vi "STS Calculator-File.vi"(6 "Hysteresis Analysis":enum32{"1st Sweep", "2nd Sweep", "Both"}(radio), 8 "NumPts":i32=3, 9 "Vd_Lin Index":i32, 10 "Vd_Sat Index":i32, 11 "Path":path) -> (0 "Used Points":T1, 1 "XY Graph-Sat":cluster{dbl[], dbl[]}[](graph), 2 "XY Graph-Lin":cluster{dbl[], dbl[]}[](graph), 3 "Ouput":cluster{"STS-Sat":dbl, "STS-Lin":dbl})   [LabVIEW 2012]
uses:
  <vilib>/Utility/file.llb/Read From Spreadsheet File (string).vi
panel:
  out "STS-Lin":dbl
  out "Linear Id":dbl[](array[numeric])
  out "Saturation Id":dbl[](array[numeric])
  out "Vg Column":dbl[](array[numeric])
  out "STS-Sat":dbl
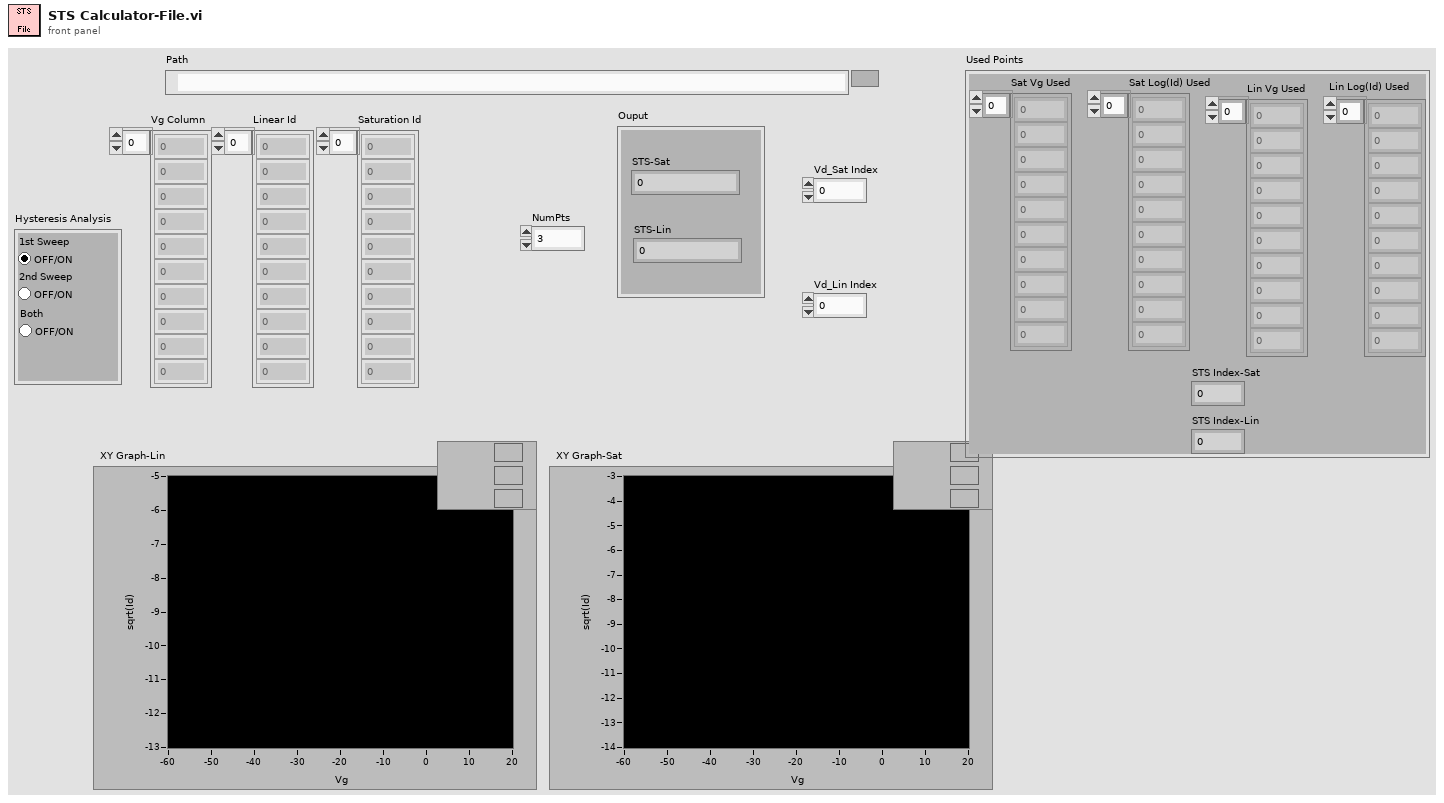
[diagram p1: front panel]
types:
  T1 = cluster{"Sat Vg Used":dbl[], "Sat Log(Id) Used":dbl[], "Lin Vg Used":dbl[], "Lin Log(Id) Used":dbl[], "STS Index-Sat":dbl, "STS Index-Lin":dbl}
  T2 = cluster{"Sub Threshold Swing":dbl, "Sub Threshold Swing":dbl}
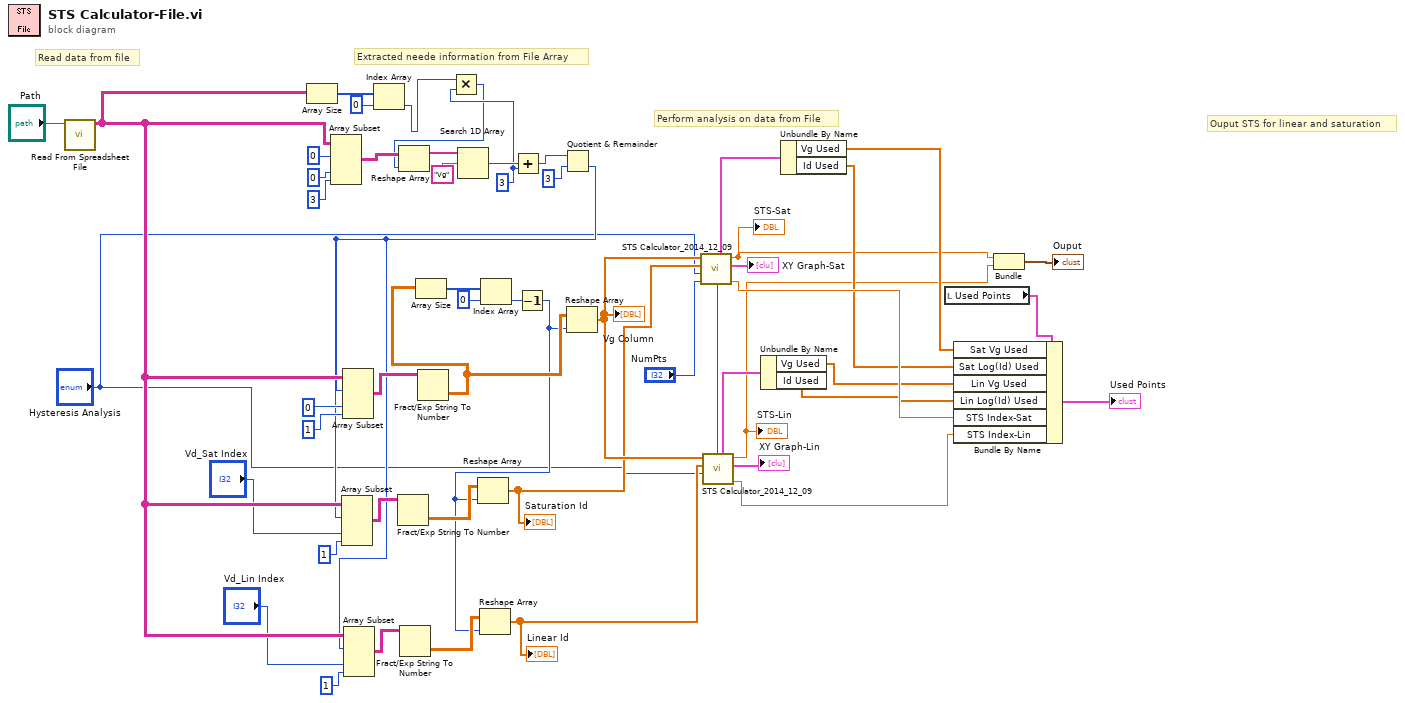
[diagram p0: block diagram]
diagram:
  w7 = 3
  # "Ouput STS for linear and saturation"
  # "Read data from file"
  # "Extracted neede information from File Array"
  # "Perform analysis on data from File"
  n1 = call-poly <vilib>:"Read From Spreadsheet File.vi"("file path (dialog if empty)"="Path") -> ("all rows"=w17:string[][])  [unwired: 6 in, 4 out]
  n2 = Array Size(array=w17) -> (size(s)=w28:i32[])
  n3 = Array Subset(array=w17, index (row)=0, index (col)=0, length (col)=3) -> (w40:string[][])  [unwired: 1 in]
  n4 = Index Array(array=w28, index=0) -> (element=w6:i32)
  n5 = Multiply(x=w6, y=w7) -> (x*y=w5:i32)
  n6 = Reshape Array(w40, w5) -> (w41:string[])
  n7 = Search 1D Array(1D array=w41, element="Vg") -> (index of element=w35:i32)  [unwired: 1 in]
  n8 = Add(x=w35, y=w7) -> (x+y=w10:i32)
  n9 = Quotient & Remainder(x=w10, y=3) -> (floor(x/y)=w8:i32)  [unwired: 1 out]
  n10 = Array Subset(array=w17, index (row)=w8, index (col)="Vd_Sat Index", length (col)=1) -> (w30:string[][])  [unwired: 1 in]
  n11 = Array Subset(array=w17, index (row)=w8, index (col)=0, length (col)=1) -> (w31:string[][])  [unwired: 1 in]
  n12 = Array Subset(array=w17, index (row)=w8, index (col)="Vd_Lin Index", length (col)=1) -> (w21:string[][])  [unwired: 1 in]
  n13 = Fract/Exp String To Number(string=w30) -> (number=w23:dbl[][])  [unwired: 3 in, 1 out]
  n14 = Fract/Exp String To Number(string=w21) -> (number=w22:dbl[][])  [unwired: 3 in, 1 out]
  n15 = Fract/Exp String To Number(string=w31) -> (number=w24:dbl[][])  [unwired: 3 in, 1 out]
  n16 = Array Size(array=w24) -> (size(s)=w27:i32[])
  n17 = Index Array(array=w27, index=0) -> (element=w25:i32)
  n18 = Decrement(x=w25) -> (x-1=w19:i32)
  n19 = Reshape Array(w23, w19) -> (w14:dbl[])
  "Saturation Id" <- w14
  n20 = Reshape Array(w22, w19) -> (w13:dbl[])
  "Linear Id" <- w13
  n21 = Reshape Array(w24, w19) -> (w15:dbl[])
  "Vg Column" <- w15
  n22 = call "STS Calculator_2014_12_09.vi"("NumPts"="NumPts", "Hysteresis Analysis"="Hysteresis Analysis", "Saturation Id"=w14, "Vg Column"=w15) -> ("STS Index"=w49:dbl, "NumPts 2"=w2:i32, "XY Graph"=→"XY Graph-Sat":cluster{dbl[], dbl[]}[], "Sub Threshold Swing"=w11:dbl, "Used Points"=w48:cluster{"Vg Used":dbl[], "Id Used":dbl[]})  [unwired: 3 in]
  "STS-Sat" <- w11
  n23 = call "STS Calculator_2014_12_09.vi"("NumPts"=w2, "Hysteresis Analysis"="Hysteresis Analysis", "Saturation Id"=w13, "Vg Column"=w15) -> ("STS Index"=w50:dbl, "XY Graph"=→"XY Graph-Lin":cluster{dbl[], dbl[]}[], "Sub Threshold Swing"=w12:dbl, "Used Points"=w45:cluster{"Vg Used":dbl[], "Id Used":dbl[]})  [unwired: 3 in, 1 out]
  "STS-Lin" <- w12
  n24 = Unbundle By Name(w45) -> ("Vg Used"=w44:dbl[], "Id Used"=w43:dbl[])
  n25 = Unbundle By Name(w48) -> ("Vg Used"=w47:dbl[], "Id Used"=w46:dbl[])
  n26 = local read "Used Points"() -> (w52:T1)
  n27 = Bundle By Name(cluster=w52, "Sat Vg Used"=w47, "Sat Log(Id) Used"=w46, "Lin Vg Used"=w44, "Lin Log(Id) Used"=w43, "STS Index-Sat"=w49, "STS Index-Lin"=w50) -> (→"Used Points":T1)
  n28 = Bundle("Sub Threshold Swing"=w11, "Sub Threshold Swing"=w12) -> (→"Ouput":T2)  [unwired: 1 in]
